vi "Write Run Time Configuration.vi"(8 "error in (no error)":errorcluster, 10 "Run Time Configuration":string, 11 "Session in":refnum<class "Plugin Session.lvclass">) -> (0 "error out":errorcluster, 3 "Session out":refnum<class "Plugin Session.lvclass">)   [LabVIEW 2021, in "CIF_InstrumentStudio Plugin SDK.lvlib" / "Plugin Session.lvclass"]
doc: "Call this VI to update the run-time configuration string for your plugin panel."
uses:
  Plugin Session.lvclass
  Plugin Session.lvclass/Plugin Session.ctl
  Read Session Id.vi
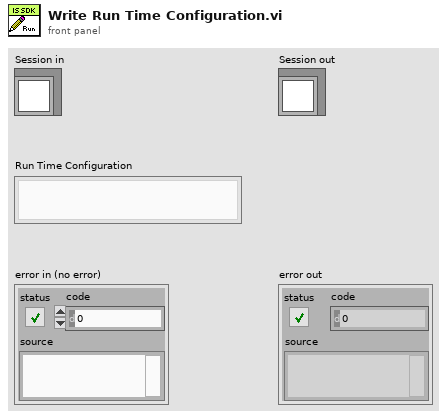
[diagram p1: front panel]
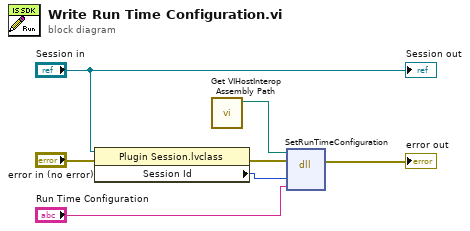
[diagram p0: block diagram]
diagram:
  n1 = property class="Plugin Session.lvclass"(reference="Session in", error in="error in (no error)") -> (error out=w7:errorcluster, "Session Id"=w6:u64)  [unwired: 1 out]
  n2 = call "Get VIHostInterop Assembly Path.vi"() -> ("VIHost.Interop Assembly"=w1:path)  [unwired: 11 in]
  n3 = dll-call lib="C:/ASW/Source/InstrumentStudio/IFDistribution/VIHostPanel/objects/export/targets/win64U/x64/msvc-14.0/debug/NationalInstruments.VIHost.Interop.dll" fn="SetRunTimeConfiguration"(path in=w1, error in=w7, "hostId"=w6, "configuration"="Run Time Configuration") -> (error out=→"error out":errorcluster)  [unwired: 4 in, 1 out]
  "Session out" <- "Session in"
